vi "Teleop.vi"(10 "Match Info":T1={"Autonomous Elapsed Seconds"=0.0, "TeleOp Elapsed Seconds"=0.0, "Disabled Elapsed Seconds"=0.0, "Visited Autonomous"=FALSE, "Visited TeleOp"=FALSE, "Visited Disabled"=FALSE, "Autonomous Settings"={"Autonomous Style"=enum."Independent", "VI Refnum"=refnum}}, 11 "Call Context":T2) -> ()   [LabVIEW 2016]
doc: "This VI is called for each TeleOp packet received from the DS where the robot is not disabled. It is often used to read from the joysticks and update I/O or to update setpoints for timed control loops. It should complete and return within 20 milliseconds or it may miss DS packets."
uses:
  <vilib>/Rock Robotics/WPI/DriverStation/WPI_DriverStationDerivedRobotMode.ctl
  <vilib>/Rock Robotics/WPI/DriverStation/WPI_DriverStationMatch Info.ctl
  <vilib>/Rock Robotics/WPI/Solenoid/WPI_SolenoidValue.ctl
  <vilib>/Rock Robotics/WPI/Utilities/WPI_GetSetVariantRefNum.vi
  <vilib>/Rock Robotics/Network Tables/NT Read Boolean.vi
  <vilib>/Rock Robotics/Network Tables/NT Read Number.vi
  <vilib>/Rock Robotics/Network Tables/NT Write Boolean.vi
  <vilib>/Rock Robotics/Network Tables/NT Write Numeric Array.vi
  <vilib>/Rock Robotics/Network Tables/NT Write Number.vi
  <vilib>/Rock Robotics/WPI/RobotDrive/WPI_RobotDriveMecanumDrive_Cartesian.vi
  Desktop/2017 Practice Code V3/2017 Steamworks Project/1-16/Documents/2017_code/Robot Global Data.vi
  <vilib>/Rock Robotics/WPI/Solenoid/WPI_SolenoidSetEnum.vi
panel:
  out "Angle":dbl(knob) scale=0.0..360.0
  out "Calibrated?":bool
  in  "Reset Angle?":bool
  out "Sample Slider 0":dbl(slide) scale=0.0..5.0
  out "Sample Boolean 1":bool
  out "Sample Boolean 0":bool
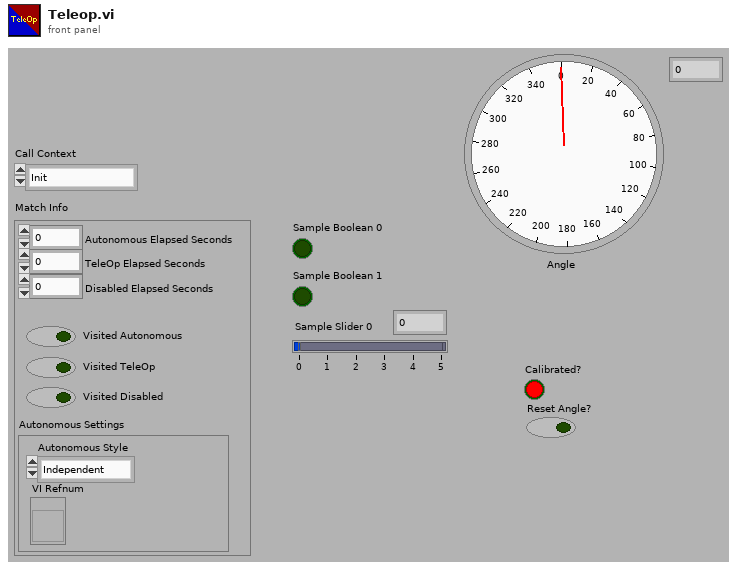
[diagram p1: front panel]
types:
  T1 = typedef "WPI_DriverStationMatch Info.ctl" = cluster{"Autonomous Elapsed Seconds":dbl, "TeleOp Elapsed Seconds":dbl, "Disabled Elapsed Seconds":dbl, "Visited Autonomous":bool, "Visited TeleOp":bool, "Visited Disabled":bool, "Autonomous Settings":cluster{"Autonomous Style":enum16{"Iterative", "Independent"}, "VI Refnum":refnum<vi>}}
  T2 = typedef "WPI_DriverStationDerivedRobotMode.ctl" = enum16{"Init", "Execute", "Stop"}
  T3 = typedef "WPI_SolenoidValue.ctl" = enum16{"Off", "On", "Forward", "Reverse"}
  T4 = typedef "WPI_RobotDriveDevRef.ctl" = cluster{"DevStatus":errorcluster, "Motors[]":T5[], "Square Inputs":bool, "Max Output":dbl}
  T5 = typedef "WPI_MotorControlDeviceRef.ctl" = cluster{"DeviceStatus":errorcluster, "Type":T6, "PWM":cluster{"PWM Channel":T7, "DeadBand":T8}, "CAN":cluster{"Device Number":u8, "SetOutput VI Ref":variant, "GetOutput VI Ref":variant, "Enable VI Ref":variant, "Disable VI Ref":variant, "Data":variant}, "Invert":bool}
  T6 = typedef "WPI_MotorControlType.ctl" = enum16{"PWM", "CAN"}
  T7 = typedef "FPGA_DIOPWMChannel.ctl" = enum8{"PWM 0", "PWM 1", "PWM 2", "PWM 3", "PWM 4", "PWM 5", "PWM 6", "PWM 7", "PWM 8", "PWM 9", "PWM MXP 0", "PWM MXP 1", "PWM MXP 2", "PWM MXP 3", "PWM MXP 4", "PWM MXP 5", "PWM MXP 6", "PWM MXP 7", "PWM MXP 8", "PWM MXP 9", "Invalid"}
  T8 = typedef "WPI_PWMDeadband.ctl" = cluster{"Name":string, "maxPositivePwm":i32, "minPositivePwm":i32, "centerPwm":i32, "maxNegativePwm":i32, "minNegativePwm":i32, "angularRange":u16}
  T9 = typedef "WPI_JoystickDevRef.ctl" = cluster{"Device":T10}
  T10 = typedef "WPI_JoystickDeviceEnum.ctl" = enum16{"USB 0", "USB 1", "USB 2", "USB 3", "USB 4", "USB 5"}
  T11 = typedef "WPI_SolenoidDevRef.ctl" = cluster{"DevStatus":errorcluster, "Pneumatics Control Module":u8, "Forward Solenoid Channel":T12, "Reverse Solenoid Channel":T12}
  T12 = typedef "WPI_SolenoidChannel.ctl" = enum8{"Solenoid 0", "Solenoid 1", "Solenoid 2", "Solenoid 3", "Solenoid 4", "Solenoid 5", "Solenoid 6", "Solenoid 7", "Invalid"}
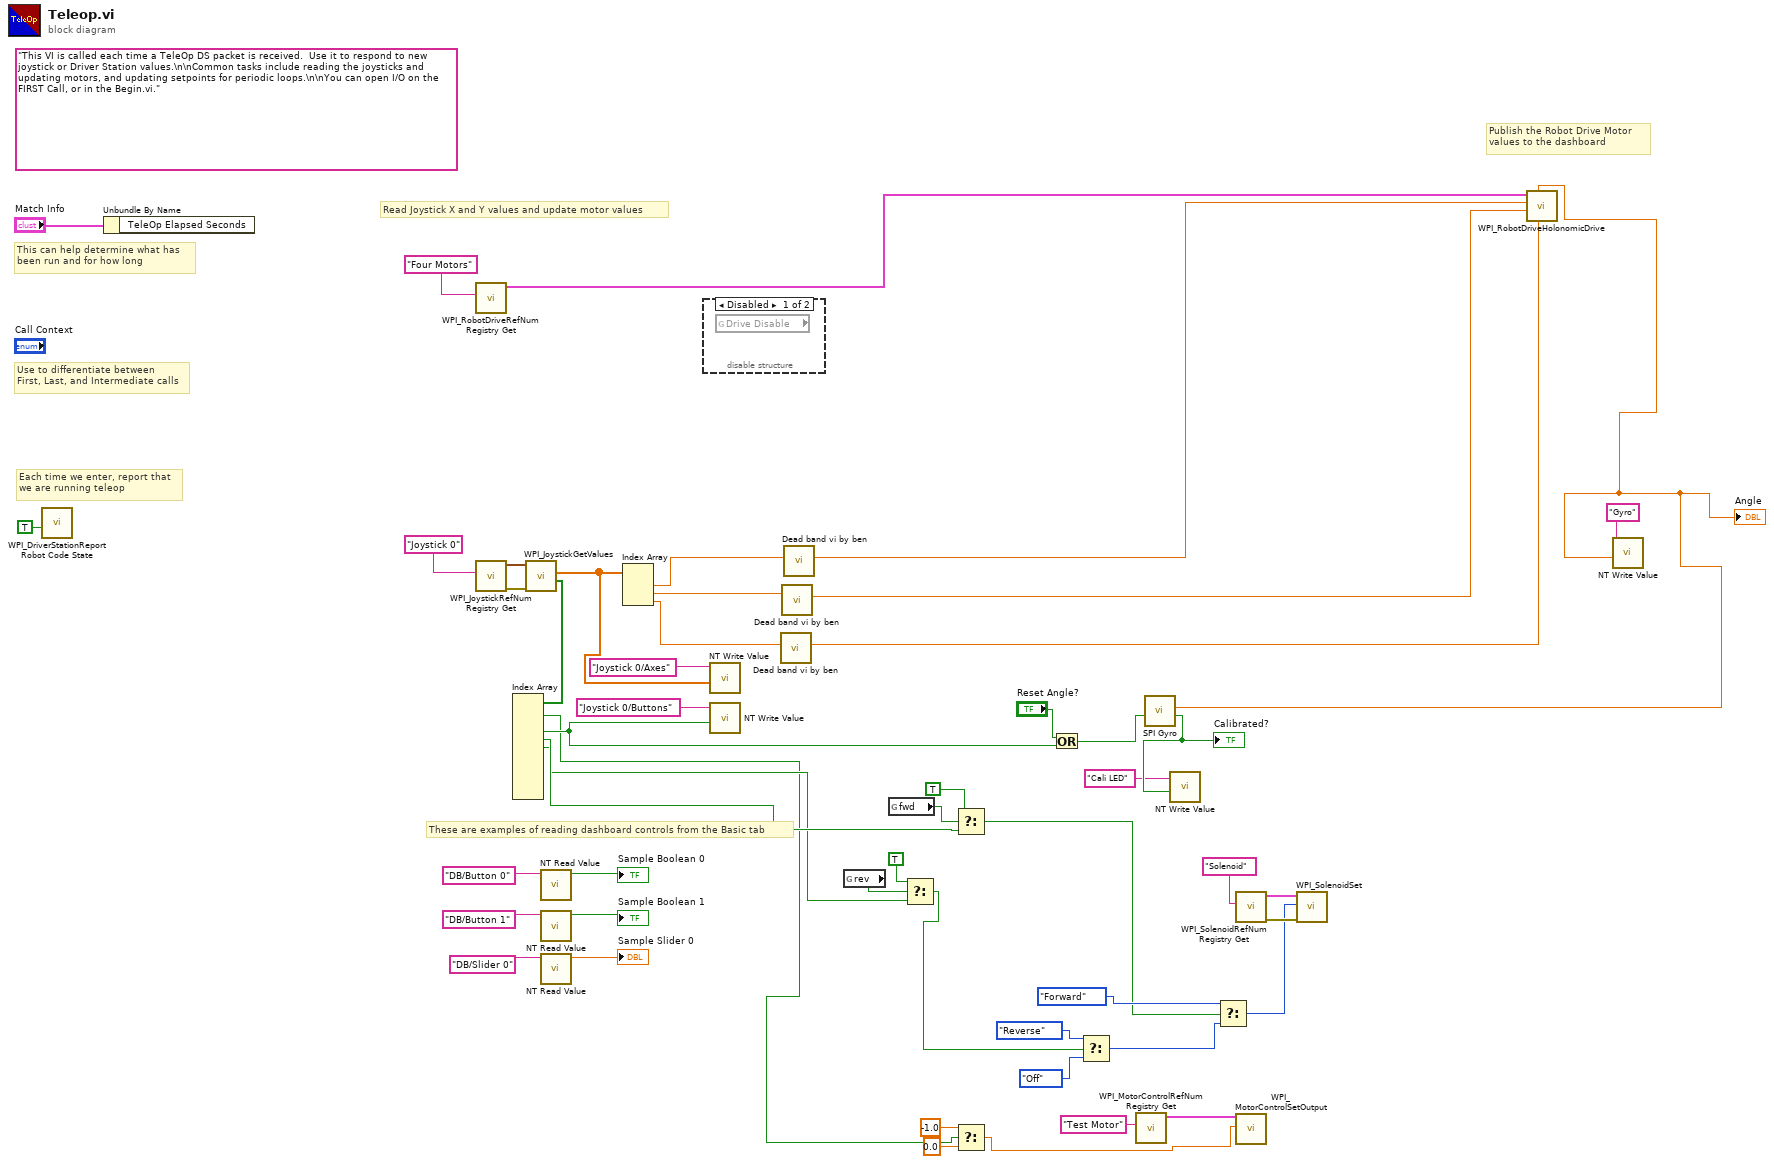
[diagram p0: block diagram]
diagram:
  (unwired) "This VI is called each time a TeleOp DS packet is received.  Use it to respond to new joystick or Driver Station values.\n\nCommon tasks include reading the joysticks and updating motors, and updating setpoints for periodic loops.\n\nYou can open I/O on the FIRST Call, or in the Begin.vi."
  # "These are examples of reading dashboard controls from the Basic tab"
  # "Publish the Robot Drive Motor\nvalues to the dashboard"
  # "Each time we enter, report that\nwe are running teleop"
  # "Use to differentiate between\nFirst, Last, and Intermediate calls"
  # "This can help determine what has\nbeen run and for how long"
  # "Read Joystick X and Y values and update motor values"
  n1 = call <vilib>:"WPI_DriverStationReport Robot Code State.vi"("TeleOp"=TRUE ("Autonomous")) -> ()  [unwired: 10 in, 1 out]
  n2 = Unbundle By Name("Match Info") -> ()  [unwired: 1 out]
  n3 = call <vilib>:"WPI_RobotDriveRefNum Registry Get.vi"("refnum name"="Four Motors") -> ("RobotDriveDevRef"=w50:T4)  [unwired: 1 in, 9 out]
  n4 = call <vilib>:"WPI_JoystickRefNum Registry Get.vi"("refnum name"="Joystick 0") -> ("error out"=w10:errorcluster, "JoystickDevRef"=w48:T9)  [unwired: 1 in, 8 out]
  n5 = call <vilib>:"WPI_JoystickGetValues.vi"("error in (no error)"=w10, "JoystickDevRef"=w48) -> ("Buttons"=w40:bool[], "Axes"=w34:dbl[])  [unwired: 5 in, 3 out]
  n6 = Index Array(array=w40) -> (element #1=w14:bool, element #3=w33:bool, element #4=w21:bool, element #5=w20:bool)  [unwired: 11 in, 7 out]
  n7 = call-poly <vilib>:"NT Read Value.vi"("Name"="DB/Button 0" ("refnum name")) -> ("Boolean"=→"Sample Boolean 0":bool)  [unwired: 9 in, 1 out]
  n8 = call-poly <vilib>:"NT Read Value.vi"("Name"="DB/Button 1" ("refnum name")) -> ("Boolean"=→"Sample Boolean 1":bool)  [unwired: 9 in, 1 out]
  n9 = call-poly <vilib>:"NT Read Value.vi"("Name"="DB/Slider 0" ("refnum name")) -> ("Numeric"=→"Sample Slider 0":dbl)  [unwired: 9 in, 1 out]
  n10 = Index Array(array=w34) -> (element #1=w39:dbl, element #2=w38:dbl, element #3=w37:dbl)  [unwired: 3 in]
  n11 = disable-structure shown="Disabled" {
    frame Disabled {
      n12 = global read "Robot Global Data.vi" "Drive Disable"() -> ()  [unwired: 1 out]
    }
    frame Enabled {
    }
  }
  n13 = call-poly <vilib>:"NT Write Value.vi"("Numeric Array"=w34, "Name"="Joystick 0/Axes") -> ()  [unwired: 9 in, 1 out]
  n14 = call-poly <vilib>:"NT Write Value.vi"("Boolean"=w33, "Name"="Joystick 0/Buttons") -> ()  [unwired: 9 in, 1 out]
  n15 = call "Dead band vi by ben.vi"("Numeric"=w37) -> ("Deadbanded Value"=w8:dbl)  [unwired: 10 in]
  n16 = call "Dead band vi by ben.vi"("Numeric"=w38) -> ("Deadbanded Value"=w9:dbl)  [unwired: 10 in]
  n17 = call "Dead band vi by ben.vi"("Numeric"=w39) -> ("Deadbanded Value"=w2:dbl)  [unwired: 10 in]
  n18 = global read "Robot Global Data.vi" "rev"() -> (w23:bool)
  n19 = global read "Robot Global Data.vi" "fwd"() -> (w24:bool)
  n20 = Select(t=TRUE, s=w23, f=w20) -> (s? t:f=w19:bool)
  n21 = Select(t=TRUE, s=w24, f=w21) -> (s? t:f=w25:bool)
  n22 = Select(t=-1.0, s=w14, f=0.0) -> (s? t:f=w11:dbl)
  n23 = Or(x="Reset Angle?", y=w33) -> (x .or. y?=w5:bool)
  n24 = Select(t=WPI_SolenoidValue."Reverse" ("Value"), s=w19, f=WPI_SolenoidValue."Off" ("Value")) -> (s? t:f=w27:T3)
  n25 = call <vilib>:"WPI_MotorControlRefNum Registry Get.vi"("refnum name"="Test Motor") -> ("MotorControlDevRef"=w16:T5)  [unwired: 9 in, 1 out]
  n26 = call "SPI Gyro.vi"("Reset"=w5) -> ("Calibrated?"=w4:bool, "Angle"=w1:dbl)  [unwired: 8 in, 1 out]
  "Angle" <- w1
  "Calibrated?" <- w4
  n27 = call-poly <vilib>:"NT Write Value.vi"("Boolean"=w4, "Name"="Cali LED") -> ()  [unwired: 9 in, 1 out]
  n28 = Select(t=WPI_SolenoidValue."Forward" ("Value"), s=w25, f=w27) -> (s? t:f=w28:T3)
  n29 = call <vilib>:"WPI_SolenoidRefNum Registry Get.vi"("refnum name"="Solenoid") -> ("error out"=w32:errorcluster, "SolenoidDevRef"=w31:T11)  [unwired: 9 in]
  n30 = call <vilib>:"WPI_MotorControlSetOutput.vi"("Output"=w11, "MotorControlDevRef"=w16) -> ()  [unwired: 7 in, 3 out]
  n31 = call-poly <vilib>:"WPI_SolenoidSet.vi"("error in (no error)"=w32, "Value"=w28, "SolenoidDevRef"=w31) -> ()  [unwired: 7 in, 2 out]
  n32 = call-poly <vilib>:"WPI_RobotDriveHolonomicDrive.vi"("Rotation"=w8, "Gyro Angle"=w1, "Y"=w9, "X"=w2, "RobotDriveDevRef"=w50) -> ()  [unwired: 4 in, 3 out]
  n33 = call-poly <vilib>:"NT Write Value.vi"("Numeric"=w1, "Name"="Gyro") -> ()  [unwired: 9 in, 1 out]
